vi "FR GUI Recalculate.vi"(10 "FR measurement":T1={"Measurement frequencies (Hz)"=[1000.0, 10000.0, 1000.0], "Sampling frequency (Hz)"=500000.0, "Signal amplitude (V)"=4.5, "AC-DC settle time (s)"=20.0, "Record length (multiples of period)"=[1000.0, 10000.0, 1000.0], "Measurement template file"=path "", "Row of START keyword"=0, "Row of STOP keyword"=0, "Calculate RMS from samples"=FALSE, "AC-DC warm up time (s)"=300.0, "Measurement template line"=[], "DC meter readings No."=10, "Algorithm"="TWM-WFFT", "Simultaneous measurement"=FALSE, "Recalculate-skip already calculated"=FALSE} {"Record length (multiples of period)" format="%#_3p"; "Sampling frequency (Hz)" format="%#_3p"; "Measurement frequencies (Hz)" format="%#_3p"}, 11 "Common properties":T2={"Measurement status ref"=refnum, "TWM Status ref"=refnum, "Abort ref"=refnum, "Skip waiting ref"=refnum, "GNU Octave path"=path "C:/Program Files/GNU Octave/Octave-6.2.0/mingw64/bin", "TWM+QWTB path"=path "C:/Users/labina/Desktop/TWM-1.8.7.0-full/octprog", "lvlib path"=path "D:/martin/WAC/WACsw - github/control_software/Filter function meter/external libraries/GOLPI 0.7.3.1 source distribution LV 20.0 32 bit/lv_proc.dll", "TWM pipe"="\\\\.\\pipe\\TWM:server", "PJVS status ref"=refnum, "WAC path"=path ""}) -> (2 "FR measurement out":T1={"Measurement frequencies (Hz)"=[1000.0, 10000.0, 1000.0], "Sampling frequency (Hz)"=500000.0, "Signal amplitude (V)"=4.5, "AC-DC settle time (s)"=20.0, "Record length (multiples of period)"=[1000.0, 10000.0, 1000.0], "Measurement template file"=path "", "Row of START keyword"=0, "Row of STOP keyword"=0, "Calculate RMS from samples"=FALSE, "AC-DC warm up time (s)"=300.0, "Measurement template line"=[], "DC meter readings No."=10, "Algorithm"="TWM-WFFT", "Simultaneous measurement"=FALSE, "Recalculate-skip already calculated"=FALSE} {"Record length (multiples of period)" format="%#_3p"; "Sampling frequency (Hz)" format="%#_3p"; "Measurement frequencies (Hz)" format="%#_3p"}, 3 "Common properties out":T2={"Measurement status ref"=refnum, "TWM Status ref"=refnum, "Abort ref"=refnum, "Skip waiting ref"=refnum, "GNU Octave path"=path "C:/Program Files/GNU Octave/Octave-6.2.0/mingw64/bin", "TWM+QWTB path"=path "C:/Users/labina/Desktop/TWM-1.8.7.0-full/octprog", "lvlib path"=path "D:/martin/WAC/WACsw - github/control_software/Filter function meter/external libraries/GOLPI 0.7.3.1 source distribution LV 20.0 32 bit/lv_proc.dll", "TWM pipe"="\\\\.\\pipe\\TWM:server", "PJVS status ref"=refnum, "WAC path"=path ""})   [LabVIEW 2020]
doc: "GUI to setup and run (re)calculation of the data obtiained during the mesurement procedure used to estimate frequency response of the digitizer."
uses:
  Utilities/Type definitions/Common properties.ctl
  FR Measurement/Type definitions/FR measuement.ctl
  <vilib>/Utility/NIReport.llb/Report Type.ctl
  <vilib>/Utility/error.llb/Error Cluster From Error Code.vi
  <vilib>/addons/_office/excel.llb/Excel Get Data ([str]).vi
  <vilib>/ErrorRing/Error Ring.xnode
  <vilib>/Utility/NIReport.llb/NI_report.lvclass
  external libraries/varilib/varilib.lvlib
  <vilib>/addons/_office/NI_ReportGenerationToolkit.lvlib
  <vilib>/Utility/NIReport.llb/NI_ReportGenerationCore.lvlib
  <vilib>/Utility/NIReport.llb/Excel/NI_Excel.lvclass
panel:
  out "template file":string
  in  "Abort":bool
  in  "skip calculated":bool caption="Skip already calculated (only rereads results)"
  out "Progress":i32(slide) min=0 max=266 scale=0.0..666.0
  out "gui_elements":refnum<vi>[](array[refnum])
  in  "OK":bool
  in  "cancel":bool
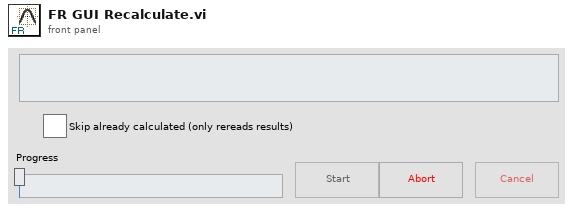
[diagram p1: front panel]
types:
  T1 = typedef "FR measuement.ctl" = cluster{"Measurement frequencies (Hz)":dbl[], "Sampling frequency (Hz)":dbl, "Signal amplitude (V)":dbl, "AC-DC settle time (s)":dbl, "Record length (multiples of period)":dbl[], "Measurement template file":path, "Row of START keyword":i32, "Row of STOP keyword":i32, "Calculate RMS from samples":bool, "AC-DC warm up time (s)":dbl, "Measurement template line":i32[], "DC meter readings No.":i32, "Algorithm":string, "Simultaneous measurement":bool, "Recalculate-skip already calculated":bool}
  T2 = typedef "Common properties.ctl" = cluster{"Measurement status ref":refnum<vi>, "TWM Status ref":refnum<vi>, "Abort ref":refnum<vi>, "Skip waiting ref":refnum<vi>, "GNU Octave path":path, "TWM+QWTB path":path, "lvlib path":path, "TWM pipe":string, "PJVS status ref":refnum<vi>, "WAC path":path}
  T3 = enum8{"Enabled", "Disabled", "Disabled and Grayed Out"}
  T4 = enum16{"maximized", "minimized", "normal", "no change"}
  T5 = typedef "NI_ReportGenerationCore.lvlib/Report Type.ctl" = enum16{"HTML", "Word", "Excel"}
  T6 = typedef "Type definitions to be saved.ctl" = cluster{"Common properties":T2, "AC Source":T7, "DC meter":T9, "CE measurement":T11, "FR measurement":T1, "FR template":T12, "CE template":T13, "PJVS":T14, "SS measurement":T18, "AC sync source":T7}
  T7 = typedef "AC Source.ctl" = cluster{"AC Source type":T8, "VISA":refnum<visa-resource-name>, "Ref. clock (Hz)":dbl, "status ref":refnum<vi>, "Fluke 57XX wideband output":bool, "Fluke 57XX ignore errors":bool, "Synchronization by AC signal":bool}
  T8 = typedef "AC Source type.ctl" = enum16{"Fluke 5XXX calibrator", "Tektronix AFG3000 series", "dummy", "Agilent 331xxA to 332xxA", "Agilent 335xxA to 336xxA"}
  T9 = typedef "DC meter.ctl" = cluster{"DC meter type":T10, "DC meter VISA":refnum<visa-resource-name>, "NPLC":dbl, "status ref":refnum<vi>}
  T10 = typedef "DC meter type.ctl" = enum16{"H/A/K 3458", "Fluke 8508A", "dummy", "Keithley 2182"}
  T11 = typedef "CE measurement.ctl" = cluster{"Signal frequencies (Hz) T":dbl[], "Signal amplitudes (V) T":dbl[], "Sampling frequencies (Hz) T":dbl[], "Record lengths (multiples of periods) T":dbl[], "TWM data root directory":path, "TWM mreasurements directories":path[], "Calculate RMS from samples":bool, "RMS algorithm T":string, "Settle down after AC source change (s) T":dbl, "Skip PJVS setup":bool, "Measurement template file":path, "Row of START keyword T":i32, "Row of STOP keyword T":i32, "Measurement template line T":i32[], "Switch position T":dbl[], "FR fit mat file T":path, "Recalculate-skip already calculated":bool}
  T12 = typedef "FR template.ctl" = cluster{"Keywords column":i32, "Sig. freq. column":i32, "Rec. len. column":i32, "Meas. points. row min to read":i32, "Meas. points. row max to read":i32, "Properties column":i32, "Properties row start":i32, "Properties row end":i32, "Keyword START regexp":string, "Keyword STOP regexp":string, "HW data column":i32, "HW data row start":i32, "HW data row end":i32, "TIme and date column start":i32, "Digitizer value column start ":i32, "DC mean column start ":i32, "DC readings column start":i32}
  T13 = typedef "CE template.ctl" = cluster{"Keywords column":i32, "Sig. freq. column":i32, "Rec. len. column":i32, "Switch pos column":i32, "Meas. points. row min to read":i32, "Meas. points. row max to read":i32, "Properties column":i32, "Properties row start":i32, "Properties row end":i32, "Keyword START regexp":string, "Keyword STOP regexp":string, "HW data column":i32, "HW data row start":i32, "HW data row end":i32, "TIme and date column start":i32, "Digitizer value column start ":i32}
  T14 = typedef "PJVS.ctl" = cluster{"PJVS type":T15, "Status Refnum":refnum<vi>, "AC-supraVOLTcontrol":cluster{"IP address:port (0.0.0.0:0000)":string, "Timeouts":T16, "Simulation mode":bool, "Debug mode":bool}, "NPL bias source":cluster{"DataSocketCluster":T17}, "Manual PJVS":cluster{"PJVS frequency (Hz)":dbl, "Reference voltages (V)":dbl[], "File with PJVS voltages":path}, "VTT PJVS":cluster{"some VTT only property":string}}
  T15 = typedef "PJVS Type.ctl" = enum16{"AC-supraVOLTcontrol", "JV modified NPL bias control", "Manual PJVS", "VTT PJVS"}
  T16 = typedef "ACSVcontrol-driver.lvlib/Timeouts.ctl" = cluster{"TCP Read & Write (ms)":i32, "Sensors readout":i32, "PJVS setup":i32, "Nullmeter readout":i32, "Multiplexer setup":i32, "57XX setup":i32, "Generator setup":i32, "Synthesizer setup":i32, "Sampler readout":i32}
  T17 = typedef "DataSocketCluster external.ctl" = cluster{"Server Machine":string, "Client Machine":string, "Data":string, "TimeStamp":dbl, "Count":i32, "Target Process":string}
  T18 = typedef "SS measurement.ctl" = cluster{"Signal frequencies (Hz)":dbl[], "Signal amplitudes (V)":dbl[], "Sampling frequencies (Hz)":dbl[], "Record lengths (multiples of periods)":dbl[], "Calculate results":bool, "Algorithm":string, "TWM data directories":path[], "TWM data directories relative":path[], "Settle down after AC source change (s)":dbl, "PJVS frequencies (Hz)":dbl[], "PJVS reference voltages array of vector cluster":cluster{"PJVS reference voltages vector":dbl[]}[], "Requested PJVS steps":u32[], "Measure CE":bool, "Measure CE before":bool, "Measure CE after":bool, "Single point CE measurement":bool, "original CE template path":path, "new CE template path before SS":path, "new CE template path before SS relative":path, "new CE template path after SS":path, "new CE template path after SS relative":path, "original CE fit path":path, "new CE fit path before SS":path, "new CE fit path before SS relative":path, "new CE fit path after SS":path, "new CE fit path after SS relative":path, "Measure digitizer gain":bool, "Measure digitizer gain before":bool, "Measure digitizer gain after":bool, "Digitizer gain":dbl, "Data folder":path, "FR fit path":path, "new FR fit path relative":path, "Rs":i32, "Re":i32, "SS measurement info files":path[]}
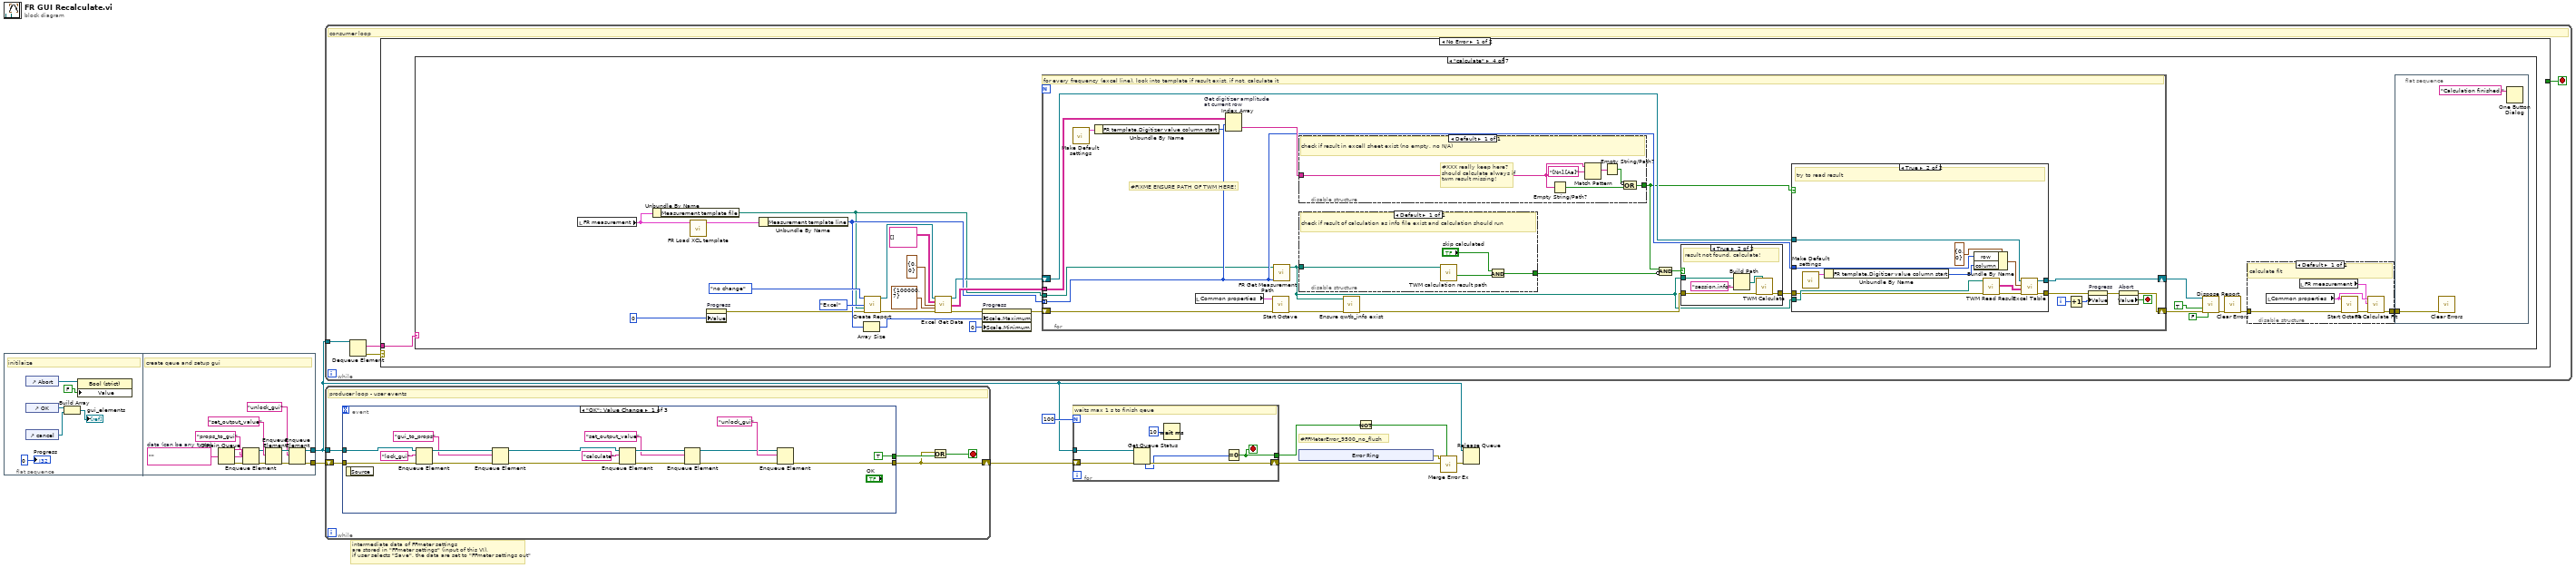
[diagram p0: block diagram]
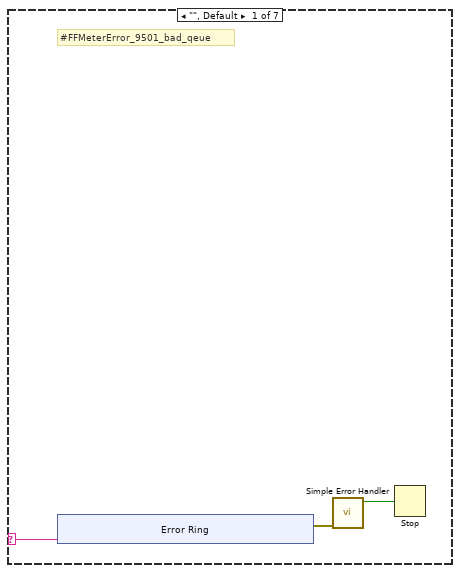
[diagram p2: hidden frame]
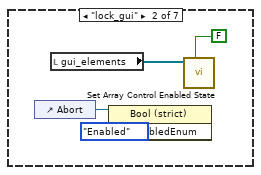
[diagram p3: hidden frame]
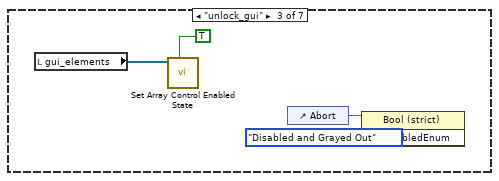
[diagram p4: hidden frame]
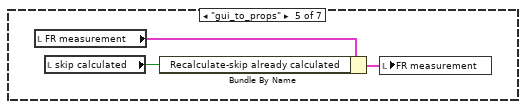
[diagram p7: hidden frame]
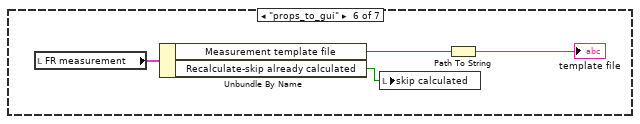
[diagram p8: hidden frame]
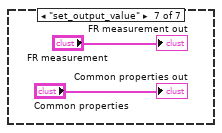
[diagram p9: hidden frame]
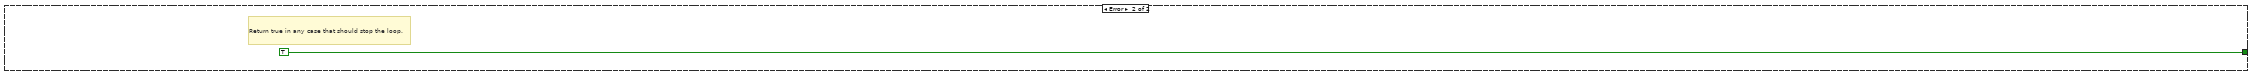
[diagram p10: hidden frame]
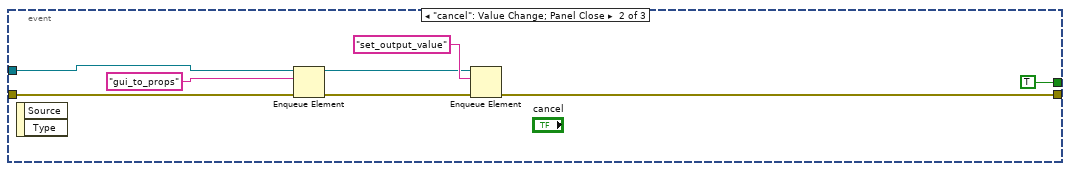
[diagram p11: hidden frame]
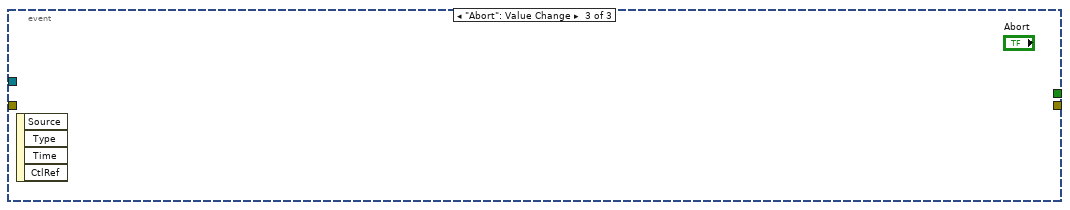
[diagram p12: hidden frame]
diagram:
  # "intermediate data of FFmeter settings\nare stored in \"FFmeter settings\" (input of this VI),\nif user selects \"Save\", the data are set to \"FFmeter settings out\""
  # "#FFMeterError_9500_no_flush"
  n1 = flat-sequence {
    tunnel: [w17] -> w2
    tunnel: [w18] -> w1
    frame #0 {
      # "initilaize"
      n2 = control-ref of="Abort"() -> (w11:refnum<vi>)
      n3 = control-ref of="OK"() -> (w15:refnum<vi>)
      n4 = control-ref of="cancel"() -> (w14:refnum<vi>)
      n5 = Build Array(w15, w14) -> (→"gui_elements":refnum<vi>[])
      n6 = property class="Bool (strict)"(reference=w11, "Value"=FALSE) -> ()  [unwired: 1 in, 2 out]
      "Progress" <- 0 ("Progress")
    }
    frame #1 {
      w26 = ""  # data (can be any type)
      # "create qeue and setup gui"
      n7 = Obtain Queue(element data type=w26) -> (queue out=w23:refnum<queue>, error out=w22:errorcluster)  [unwired: 4 in, 1 out]
      n8 = Enqueue Element(queue=w23, element="props_to_gui", error in (no error)=w22) -> (queue out=w24:refnum<queue>, error out=w25:errorcluster)  [unwired: 1 in, 1 out]
      n9 = Enqueue Element(queue=w24, element="set_output_value", error in (no error)=w25) -> (queue out=w20:refnum<queue>, error out=w19:errorcluster)  [unwired: 1 in, 1 out]
      n10 = Enqueue Element(queue=w20, element="unlock_gui", error in (no error)=w19) -> (queue out=w17:refnum<queue>, error out=w18:errorcluster)  [unwired: 1 in, 1 out]
    }
  }
  n11 = while {
    tunnel: w2 -> [w31]
    stop <- w28 stop-if-true
    # "consumer loop"
    n12 = Dequeue Element(queue=w31) -> (element=w29:string, error out=w30:errorcluster)  [unwired: 2 in, 2 out]
    n13 = case shown="No Error" w30 {
      tunnel: w29 -> [w32 _]
      tunnel: [_ TRUE] -> w28
      frame No Error {
        n14 = case shown="\"calculate\"" w32 {
          selector: w32 -> [w33 _ _ _ _ _ _]
          frame "", Default {
            # "#FFMeterError_9501_bad_qeue"
            n15 = xnode "Error Ring"("parameter 0"=w33) -> ("error out"=w35:errorcluster)
            n16 = call <vilib>:"Simple Error Handler.vi"("error in (no error)"=w35) -> ("error?"=w34:bool)  [unwired: 4 in, 4 out]
            n17 = Stop(stop? (T)=w34) -> ()
          }
          frame "lock_gui" {
            n18 = control-ref of="Abort"() -> (w44:refnum<vi>)
            n19 = local read "gui_elements"() -> (w46:refnum<vi>[])
            n20 = property class="Bool (strict)"(reference=w44, "DisabledEnum"=T3."Enabled" ("Disabled")) -> ()  [unwired: 1 in, 2 out]
            n21 = call "Set Array Control Enabled State.vi"("enabled (T)"=FALSE, "reference array in"=w46) -> ()  [unwired: 8 in, 2 out]
          }
          frame "unlock_gui" {
            n22 = local read "gui_elements"() -> (w50:refnum<vi>[])
            n23 = call "Set Array Control Enabled State.vi"("enabled (T)"=TRUE, "reference array in"=w50) -> ()  [unwired: 8 in, 2 out]
            n24 = control-ref of="Abort"() -> (w47:refnum<vi>)
            n25 = property class="Bool (strict)"(reference=w47, "DisabledEnum"=T3."Disabled and Grayed Out" ("Disabled")) -> ()  [unwired: 1 in, 2 out]
          }
          frame "calculate" {
            n26 = local read "FR measurement"() -> (w55:T1)
            n27 = Unbundle By Name(w55) -> ("Measurement template file"=w54:path)
            n28 = call "FR Load XCL template.vi"("FR measurement"=w55) -> ("FR measurement out"=w69:T1)  [unwired: 10 in]
            n29 = property on="Progress" class="Slide (strict)"("Value"=0 ("Progress")) -> (error out=w65:errorcluster)  [unwired: 2 in, 1 out]
            n30 = Unbundle By Name(w69) -> ("Measurement template line"=w67:i32[])
            n31 = Array Size(array=w67) -> (size(s)=w66:i32)
            n32 = call <vilib>:"Create Report.vi"("window state (normal)"=T4."no change", "report type"=Report_Type."Excel", "template (empty)"=w54, "error in (no error)"=w65) -> ("report out"=w70:refnum<class "NI_report.lvclass">, "error out"=w71:errorcluster)  [unwired: 10 in]
            n33 = call-poly <vilib>:"Excel Get Data.vi"("report in"=w70, "data type"=string[][] [], "start (-1, -1)"=cluster{"row":i32, "column":i32} {"row"=0, "column"=0}, "end (-1, -1)"=cluster{"row":i32, "column":i32} {"row"=100000, "column"=7}, "error in (no error)"=w71) -> ("report out"=w63:refnum<class "NI_report.lvclass">, "data"=w68:string[][], "error out"=w62:errorcluster)  [unwired: 8 in]
            n34 = property on="Progress" class="Slide (strict)"(error in=w62, "Scale.Maximum"=w66, "Scale.Minimum"=0 ("Data Entry Limits:Minimum")) -> (error out=w61:errorcluster)  [unwired: 1 in, 1 out]
            n35 = for {
              tunnel: w67 -> [w102] mode=indexing
              shift-right: [w88] -> w58
              shift-left: w61 -> [w101]
              tunnel: w68 -> [w106]
              shift-right: [w95] -> w59
              shift-left: w63 -> [w103]
              tunnel: w54 -> [w87]
              i -> [w104]
              stop <- w89 stop-if-true
              # "#FIXME ENSURE PATH OF TWM HERE!"
              # "for every frequency (excel line), look into template if result exist. if not, calculate it"
              n36 = call "Make Default settings.vi"() -> ("TD to be saved"=w86:T6)  [unwired: 11 in]
              n37 = Unbundle By Name(w86) -> ("FR template.Digitizer value column start"=w85:i32)
              n38 = local read "Common properties"() -> (w84:T2)
              n39 = Index Array "Get digitizer amplitude\nat current row"(array=w106, index (row)=w102, index (col)=w85) -> (element=w105:string)
              n40 = call "Start Octave.vi"("error in (no error)"=w101, "Common properties"=w84) -> ("error out"=w99:errorcluster)  [unwired: 9 in]
              n41 = call "FR Get Measurement Path.vi"("Template line"=w102, "Measurement template file"=w87) -> ("Measurement path"=w92:path)  [unwired: 8 in, 1 out]
              n42 = disable-structure shown="Default" {
                disable-tunnel: w105 -> [w135]
                disable-tunnel: [w131] -> w93
                frame Enabled {
                  # "#XXX really keep here?\nshould calculate always if\ntwm result missing!"
                  # "check if result in excell sheet exist (no empty, no N/A)"
                  n43 = Empty String/Path?(string/path=w135) -> (empty?=w132:bool)
                  n44 = Match Pattern(string=w135, regular expression="[Nn].[Aa]") -> (match substring=w134:string)  [unwired: 1 in, 3 out]
                  n45 = Empty String/Path?(string/path=w134) -> (empty?=w133:bool)
                  n46 = Compound Arithmetic op=OR(invert w133, w132) -> (w131:bool)
                }
              }
              n47 = disable-structure shown="Default" {
                disable-tunnel: w92 -> [w124]
                disable-tunnel: [w121] -> w91
                frame Enabled {
                  # "check if result of calculation as info file exist and calculation should run"
                  n48 = call "TWM calculation result path.vi"("Measurement path"=w124) -> ("file exists?"=w122:bool)  [unwired: 9 in, 1 out]
                  n49 = Compound Arithmetic op=AND("skip calculated", w122) -> (w121:bool)
                }
              }
              n50 = call "Ensure qwtb_info exist.vi"("error in"=w99, "Measurement path"=w92) -> ("error out"=w98:errorcluster)  [unwired: 9 in]
              n51 = Compound Arithmetic op=AND(w93, invert w91) -> (w97:bool)
              n52 = case shown="True" w97 {
                tunnel: w98 -> [w125 w130]
                tunnel: [w125 w129] -> w94
                tunnel: w92 -> [_ w127]
                frame False {
                  # "result existr"
                }
                frame True {
                  # "result not found, calculate!"
                  n53 = Build Path(base path=w127, name or relative path="session.info") -> (appended path=w126:path)
                  n54 = call "TWM Calculate.vi"("session info path"=w126, "error in (no error)"=w130) -> ("error out"=w129:errorcluster)  [unwired: 9 in]
                }
              }
              n55 = case shown="True" w93 {
                tunnel: w103 -> [w107 w120]
                tunnel: w102 -> [_ w119]
                tunnel: w92 -> [_ w118]
                tunnel: [w108 w117] -> w96
                tunnel: [w107 w116] -> w95
                tunnel: w94 -> [w108 w113]
                frame False {
                }
                frame True {
                  # "try to read result"
                  n56 = call "Make Default settings.vi"() -> ("TD to be saved"=w110:T6)  [unwired: 11 in]
                  n57 = Unbundle By Name(w110) -> ("FR template.Digitizer value column start"=w109:i32)
                  n58 = Bundle By Name(cluster=cluster{"row":i32, "column":i32} {"row"=0, "column"=0} ("start (0, 0)"), "row"=w119, "column"=w109) -> (w114:cluster{"row":i32, "column":i32})
                  n59 = call "TWM Read Result.vi"("error in (no error)"=w113, "Measurement path"=w118) -> ("error out"=w112:errorcluster, "Result (val, unc)"=w111:string[][])  [unwired: 8 in]
                  n60 = call "Excel Table.vi"("error in (no error)"=w112, "table"=w111, "start (0, 0)"=w114, "report in"=w120) -> ("error out"=w117:errorcluster, "report out"=w116:refnum<class "NI_report.lvclass">)  [unwired: 6 in]
                }
              }
              n61 = Increment(x=w104) -> (x+1=w100:i32)
              n62 = property on="Progress" class="Slide (strict)"(error in=w96, "Value"=w100) -> (error out=w90:errorcluster)  [unwired: 1 in, 1 out]
              n63 = property on="Abort" class="Bool (strict)"(error in=w90) -> (error out=w88:errorcluster, "Value"=w89:bool)  [unwired: 1 in, 1 out]
            }
            n64 = call-dynamic "Dispose Report.vi"("report in"=w59, "save changes? (F)"=TRUE, "error in (no error)"=w58, "close report? (T)"=FALSE) -> ("error out"=w53:errorcluster)  [unwired: 11 in]
            n65 = call <vilib>:"Clear Errors.vi"("error in (no error)"=w53) -> ("error out"=w52:errorcluster)  [unwired: 5 in, 1 out]
            n66 = disable-structure shown="Default" {
              disable-tunnel: w52 -> [w81]
              disable-tunnel: [w79] -> w51
              frame Enabled {
                # "calculate fit"
                n67 = local read "Common properties"() -> (w78:T2)
                n68 = local read "FR measurement"() -> (w77:T1)
                n69 = call "Start Octave.vi"("error in (no error)"=w81, "Common properties"=w78) -> ("error out"=w80:errorcluster)  [unwired: 9 in]
                n70 = call "FR Calculate Fit.vi"("error in (no error)"=w80, "FR measurement"=w77, "Common properties"=w78) -> ("error out"=w79:errorcluster)  [unwired: 8 in]
              }
            }
            n71 = flat-sequence {
              tunnel: w51 -> [w82]
              frame #0 {
                n72 = call <vilib>:"Clear Errors.vi"("error in (no error)"=w82) -> ()  [unwired: 5 in, 2 out]
                n73 = One Button Dialog(message="Calculation finished.") -> ()  [unwired: 1 in, 1 out]
              }
            }
          }
          frame "gui_to_props" {
            n74 = local read "FR measurement"() -> (w139:T1)
            n75 = local read "skip calculated"() -> (w138:bool)
            n76 = Bundle By Name(cluster=w139, "Recalculate-skip already calculated"=w138) -> (w137:T1)
            n77 = local write "FR measurement"(w137) -> ()
          }
          frame "props_to_gui" {
            n78 = local read "FR measurement"() -> (w142:T1)
            n79 = Unbundle By Name(w142) -> ("Measurement template file"=w140:path, "Recalculate-skip already calculated"=w141:bool)
            n80 = local write "skip calculated"(w141) -> ()
            n81 = Path To String(path=w140) -> (string=→"template file":string)
          }
          frame "set_output_value" {
            "Common properties out" <- "Common properties"
            "FR measurement out" <- "FR measurement"
          }
        }
      }
      frame Error {
        # "Return true in any case that should stop the loop."
      }
    }
  }
  n82 = while {
    shift-right: [w147] -> w5
    shift-left: w1 -> [w150]
    tunnel: w2 -> [w151]
    stop <- w148 stop-if-true
    # "producer loop - user events"
    n83 = event shown="[0] \"OK\": Value Change" {
      selector: _ -> [_ _ _]
      dyn-events: _ -> [_ _ _]
      timeout: _ -> [_ _ _]
      tunnel: w151 -> [w166 w170 _]
      tunnel: w150 -> [w165 w173 _]
      tunnel: [w163 w174 _] -> w147
      tunnel: [TRUE ("cancel") TRUE ("cancel") _] -> w149
      event "OK": Value Change {
        n84 = event-data() -> ()  [unwired: 1 in, 1 out]
        n85 = Enqueue Element(queue=w166, element="lock_gui", error in (no error)=w165) -> (queue out=w160:refnum<queue>, error out=w162:errorcluster)  [unwired: 1 in, 1 out]
        n86 = Enqueue Element(queue=w160, element="gui_to_props", error in (no error)=w162) -> (queue out=w154:refnum<queue>, error out=w161:errorcluster)  [unwired: 1 in, 1 out]
        n87 = Enqueue Element(queue=w154, element="calculate", error in (no error)=w161) -> (queue out=w155:refnum<queue>, error out=w158:errorcluster)  [unwired: 1 in, 1 out]
        n88 = Enqueue Element(queue=w155, element="set_output_value", error in (no error)=w158) -> (queue out=w156:refnum<queue>, error out=w157:errorcluster)  [unwired: 1 in, 1 out]
        n89 = Enqueue Element(queue=w156, element="unlock_gui", error in (no error)=w157) -> (error out=w163:errorcluster)  [unwired: 1 in, 2 out]
      }
      event "cancel": Value Change; Panel Close {
        n90 = event-data() -> ()  [unwired: 1 in, 2 out]
        n91 = Enqueue Element(queue=w170, element="gui_to_props", error in (no error)=w173) -> (queue out=w171:refnum<queue>, error out=w172:errorcluster)  [unwired: 1 in, 1 out]
        n92 = Enqueue Element(queue=w171, element="set_output_value", error in (no error)=w172) -> (error out=w174:errorcluster)  [unwired: 1 in, 2 out]
      }
      event "Abort": Value Change {
        n93 = event-data() -> ()  [unwired: 1 in, 4 out]
      }
    }
    n94 = Or(x=w147, y=w149) -> (x .or. y?=w148:bool)
  }
  n95 = for {
    N: 100 -> [_]
    tunnel: w2 -> [w182]
    shift-right: [w180] -> w6
    shift-left: w5 -> [w181]
    tunnel: [w177] -> w3
    stop <- w177 stop-if-true
    # "waits max 1 s to finish qeue"
    n96 = Get Queue Status(queue=w182, error in (no error)=w181) -> (error out=w180:errorcluster, # elements in queue=w178:i32)  [unwired: 1 in, 6 out]
    n97 = Wait (ms)(milliseconds to wait=u32 10) -> ()  [unwired: 1 out]
    n98 = Equal To 0?(x=w178) -> (x = 0?=w177:bool)
  }
  n99 = xnode "Error Ring"() -> ("error out"=w7:errorcluster)
  n100 = Not(x=w3) -> (.not. x?=w8:bool)
  n101 = call "Merge Error Ex.vi"("Is error? (False)"=w8, "main error in (no error)"=w6, "second error in"=w7) -> ("error out"=w4:errorcluster)  [unwired: 8 in]
  n102 = Release Queue(queue=w2, error in (no error)=w4) -> ()  [unwired: 1 in, 3 out]
